vi "Get Error Code from Text.vi"(8 "error in (no error)":errorcluster, 11 "text":string) -> (0 "error out":errorcluster, 2 "found?":bool, 3 "code":i32)   [LabVIEW 2016]
uses:
  <vilib>/regexp/Match Regular Expression.xnode
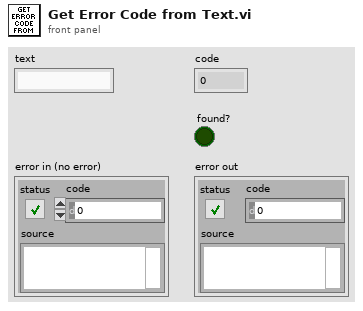
[diagram p1: front panel]
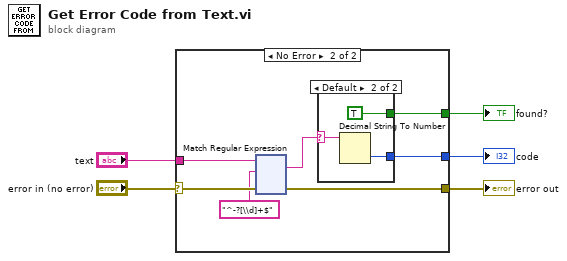
[diagram p0: block diagram]
diagram:
  n1 = case shown="No Error" "error in (no error)" {
    selector: "error in (no error)" -> [w6 w13]
    tunnel: "text" -> [_ w11]
    tunnel: [w6 w9] -> w3
    tunnel: [_ w8] -> w2
    tunnel: [_ w7] -> w1
    frame Error {
    }
    frame No Error {
      n2 = xnode "Match Regular Expression"("input string"=w11, "regular expression"="^-?[\\d]+$", "error in"=w13) -> ("whole match"=w12:string, "error out"=w9:errorcluster)  [unwired: 3 in, 3 out]
      n3 = case shown="Default" w12 {
        selector: w12 -> [_ w16]
        tunnel: [_ w15] -> w8
        tunnel: [_ TRUE] -> w7
        frame "" {
        }
        frame Default {
          n4 = Decimal String To Number(string=w16) -> (number=w15:i32)  [unwired: 2 in, 1 out]
        }
      }
    }
  }
  "error out" <- w3
  "code" <- w2
  "found?" <- w1
